vi "Glimpse display gain-offset old.vi"(4 "White level":dbl=255.0 format="%.2f", 5 "Black level":dbl format="%.2f", 6 "Pixel depth":u32, 7 "Window Number (0...15)":i32, 8 "error in":errorcluster, 9 "Resize to Image Size? (Y)":bool=TRUE, 10 "Window Title":string, 11 "Image In":T1) -> (0 "error out":errorcluster, 3 "Image Out":T1)   [LabVIEW 2016]
uses:
  <vilib>/vision/Image Controls.llb/IMAQ Image.ctl
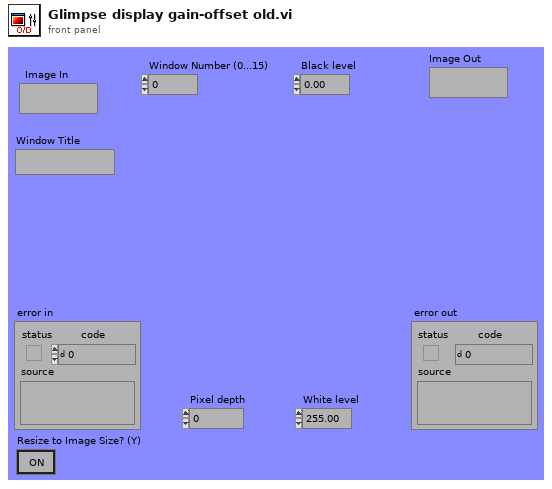
[diagram p1: front panel]
types:
  T1 = typedef "IMAQ Image.ctl" = refnum<image>
  T2 = cluster{"Conversion Method":u32, "Minimum Value":i32, "Maximum Value":i32, "# Shifts":i32}
  T3 = cluster{"upper limit":dbl, "upper limit":dbl, "upper limit":dbl}
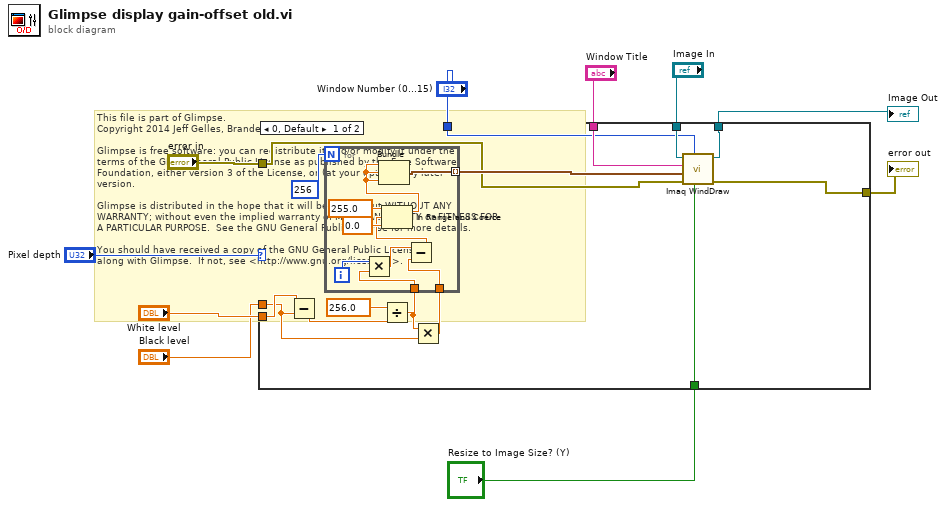
[diagram p0: block diagram]
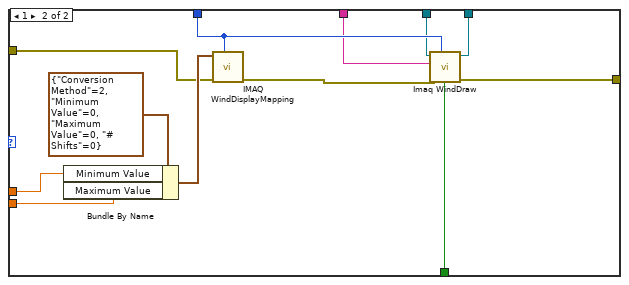
[diagram p2: hidden frame]
diagram:
  # "This file is part of Glimpse. \nCopyright 2014 Jeff Gelles, Brandeis University.    \n\nGlimpse is free software: you can redistribute it and/or modify it under the \nterms of the GNU General Public License as published by the Free Software \nFoundation, either version 3 of the License, or (at your option) any later \nversion.\n\nGlimpse is distributed in the hope that it will be useful, but WITHOUT ANY \nWARRANTY; without even the implied warranty of MERCHANTABILITY or FITNESS FOR \nA PARTICULAR PURPOSE.  See the GNU General Public License for more details.\n\nYou should have received a copy of the GNU General Public License\nalong with Glimpse.  If not, see <http://www.gnu.org/licenses/>."
  n1 = case shown="0, Default" "Pixel depth" {
    tunnel: "Window Number (0...15)" -> [w14 w39]
    tunnel: "Black level" -> [w15 w44]
    tunnel: "White level" -> [w16 w43]
    tunnel: "error in" -> [w12 w42]
    tunnel: [w13 w40] -> w7
    tunnel: "Window Title" -> [w19 w38]
    tunnel: "Image In" -> [w18 w37]
    tunnel: [w17 w36] -> w4
    tunnel: "Resize to Image Size? (Y)" -> [w11 w35]
    frame 0, Default {
      n2 = Subtract(x=w16, y=w15) -> (x-y=w23:dbl)
      n3 = Divide(x=256.0, y=w23) -> (x/y=w22:dbl)
      n4 = Multiply(x=w22, y=w15) -> (x*y=w21:dbl)
      n5 = for {
        N: 256 -> [_]
        tunnel: w22 -> [w33]
        tunnel: w21 -> [w32]
        tunnel: [w26] -> w20 mode=indexing
        i -> [w34]
        n6 = Multiply(x=w34, y=w33) -> (x*y=w31:dbl)
        n7 = Subtract(x=w31, y=w32) -> (x-y=w28:dbl)
        n8 = In Range and Coerce(upper limit=255.0, x=w28, lower limit=0.0) -> (coerced(x)=w27:dbl)  [unwired: 1 out]
        n9 = Bundle("upper limit"=w27, "upper limit"=w27, "upper limit"=w27) -> (w26:T3)  [unwired: 1 out]
      }
      n10 = call "Imaq WindDraw"("Resize to Image Size? (Y)"=w11, "Window Number (0...15)"=w14, "error in (no error)"=w12, "Color Palette"=w20, "Title"=w19, "Image"=w18) -> ("error out"=w13:errorcluster, "Image Out (duplicate)"=w17:T1)  [unwired: 4 out]
    }
    frame 1 {
      n11 = Bundle By Name(cluster=T2 {"Conversion Method"=2, "Minimum Value"=0, "Maximum Value"=0, "# Shifts"=0} ("Conversion Policy (Full Dynamic)"), "Minimum Value"=w44, "Maximum Value"=w43) -> (w45:T2)
      n12 = call "IMAQ WindDisplayMapping"("Window Number (0...15)"=w39, "error in (no error)"=w42, "Conversion Policy (Default)"=w45) -> ("error out"=w41:errorcluster)  [unwired: 1 in, 7 out]
      n13 = call "Imaq WindDraw"("Resize to Image Size? (Y)"=w35, "Window Number (0...15)"=w39, "error in (no error)"=w41, "Title"=w38, "Image"=w37) -> ("error out"=w40:errorcluster, "Image Out (duplicate)"=w36:T1)  [unwired: 1 in, 4 out]
    }
  }
  "error out" <- w7
  "Image Out" <- w4
